vi "LocalisationFileLoader.vi"(10 "error in":errorcluster, 11 "FilePath":path) -> (2 "error out":errorcluster, 3 "LocalisationFileContent[out]":T1)   [LabVIEW 2013]
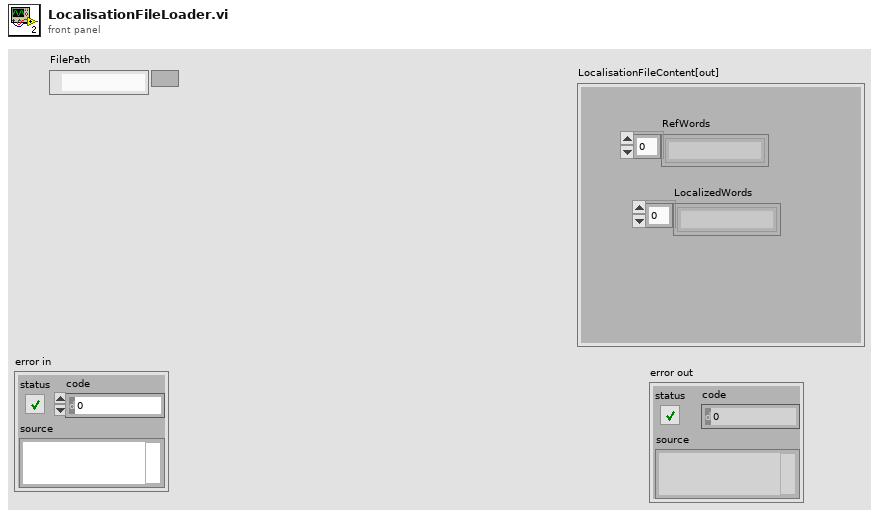
[diagram p1: front panel]
types:
  T1 = cluster{"RefWords":string[], "LocalizedWords":string[]}
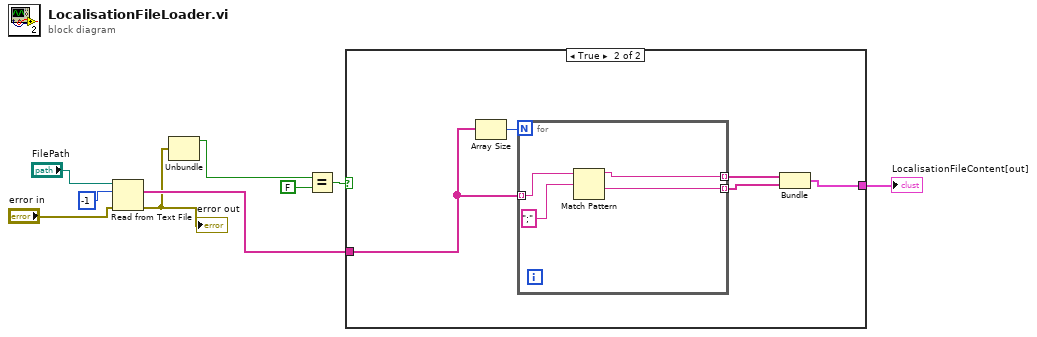
[diagram p0: block diagram]
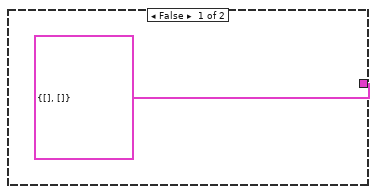
[diagram p2: hidden frame]
diagram:
  n1 = Read from Text File(file (use dialog)="FilePath", count=-1, error in="error in") -> (text=w8:string[], error out=w5:errorcluster)  [unwired: 1 in, 2 out]
  "error out" <- w5
  n2 = Unbundle(w5) -> ("status"=w3:bool)  [unwired: 2 out]
  n3 = Equal?(x=w3, y=FALSE) -> (x = y?=w4:bool)
  n4 = case shown="True" w4 {
    tunnel: w8 -> [_ w14]
    tunnel: [cluster{string[], string[]} {[], []} w11] -> w1
    frame False {
    }
    frame True {
      n5 = Array Size(array=w14) -> (size(s)=w15:i32)
      n6 = for {
        N: w15 -> [_]
        tunnel: w14 -> [w19] mode=indexing
        tunnel: [w17] -> w13 mode=indexing
        tunnel: [w16] -> w12 mode=indexing
        n7 = Match Pattern(string=w19, regular expression=";") -> (before substring=w17:string, after substring=w16:string)  [unwired: 1 in, 2 out]
      }
      n8 = Bundle(w13, w12) -> (w11:cluster{string[], string[]})  [unwired: 1 in]
    }
  }
  "LocalisationFileContent[out]" <- w1
